vi "DeInit.vi"(8 "error in (no error)":errorcluster, 11 "KIM101 in":refnum<class "KIM101.lvclass">) -> (0 "error out":errorcluster, 3 "KIM101 out":refnum<class "KIM101.lvclass">)   [LabVIEW 2023, in "KIM101.lvlib" / "KIM101.lvclass"]
uses:
  KIM101.lvclass
  C:/Program Files/National Instruments/LabVIEW 2023/vi.lib/ActorFramework/Actor/Actor.lvclass
  typedefs/instrumentType.ctl
  <vilib>/ActorFramework/Actor/Actor.lvclass/Actor.ctl
  KIM101.lvclass/KIM101.ctl
  Interfaces/InitDeinitInterface/InitDeinitComm Messages/DeInit Done Msg/DeInit Done Msg.lvclass/DeInit Done Msg.ctl
  <vilib>/ActorFramework/Message Enqueuer/Message Enqueuer.lvclass/Message Enqueuer.ctl
  <vilib>/ActorFramework/Message Enqueuer/Enqueue.vi
  Interfaces/InitDeinitInterface/InitDeinitComm Messages/DeInit Done Msg/DeInit Done Msg.lvclass
  C:/Program Files/National Instruments/LabVIEW 2023/vi.lib/ActorFramework/Message/Message.lvclass
  C:/Users/quantum/Documents/LVDAQ/UIs/TranslationStage_UI/Thorlabs.MotionControl.KCube.InertialMotorCLI.dll
  UIs/TranslationStage_UI/Thorlabs.MotionControl.KCube.InertialMotorCLI.dll
  <vilib>/ActorFramework/Message Priority Queue/Priority Enqueue.vi
  <vilib>/ActorFramework/Actor/Actor.lvclass
  <vilib>/ActorFramework/Message Enqueuer/Message Enqueuer.lvclass
  typedefs/typedefs.lvlib
panel:
  out "output cluster":T2
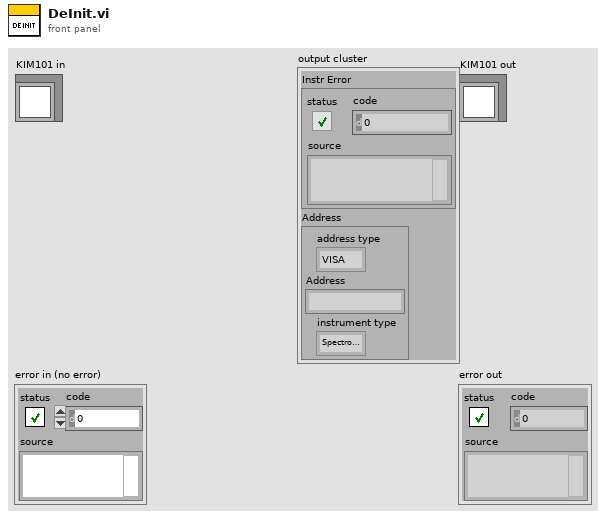
[diagram p1: front panel]
types:
  T1 = typedef "typedefs.lvlib/instrumentType.ctl" = enum16{"Spectrometer", "Camera", "Stepper", "Piezo"}
  T2 = cluster{"Instr Error":errorcluster, "Address":cluster{"address type":enum16{"VISA", "Index"}, "Address":string, "instrument type":T1}}
  T3 = cluster{"address type":enum16{"VISA", "Index"}, "Address":string, "instrument type":T1}
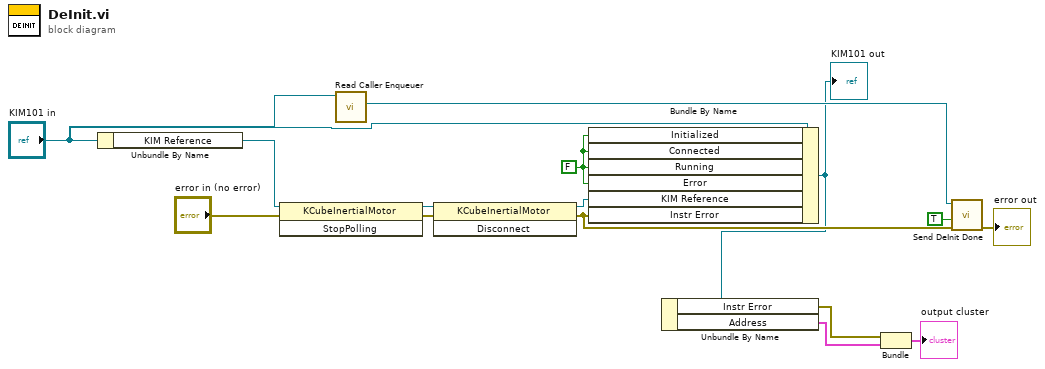
[diagram p0: block diagram]
diagram:
  w11 = FALSE ("InstrumentData.CurrentState.Error")
  n1 = Unbundle By Name("KIM101 in") -> ("KIM Reference"=w15:refnum<k24>)
  n2 = invoke class="KCubeInertialMotor" method="StopPolling"(reference=w15, error in="error in (no error)") -> (reference out=w13:refnum<k24>, error out=w12:errorcluster)  [unwired: 1 in, 1 out]
  n3 = call <vilib>:"Read Caller Enqueuer.vi"("Actor"="KIM101 in") -> ("Caller Enqueuer"=w9:refnum<class "Message Enqueuer.lvclass">)  [unwired: 10 in]
  n4 = invoke class="KCubeInertialMotor" method="Disconnect"(reference=w13, error in=w12) -> (reference out=w10:refnum<k24>, error out=w7:errorcluster)  [unwired: 1 in, 1 out]
  n5 = Bundle By Name(cluster="KIM101 in", "Initialized"=w11, "Connected"=w11, "Running"=w11, "Error"=w11, "KIM Reference"=w10, "Instr Error"=w7) -> (w5:refnum<class "KIM101.lvclass">)
  "KIM101 out" <- w5
  n6 = Unbundle By Name(w5) -> ("Instr Error"=w4:errorcluster, "Address"=w3:T3)
  n7 = Bundle("Instr Error"=w4, "Address"=w3) -> (→"output cluster":T2)  [unwired: 1 in]
  n8 = call "Send DeInit Done.vi"("error in (no error)"=w7, "Initialized"=TRUE, "Message Enqueuer"=w9) -> ("error out"=→"error out":errorcluster)  [unwired: 7 in, 1 out]
